vi "Step Make.vi"(8 "error in (no error)":errorcluster, 9 "Step Type (0: UP)":u16(ring) items=["Up", "Down"], 10 "Function (0: Voltage)":u16(ring) items=["Voltage", "Current"], 11 "VISA resource name":refnum<visa-resource-name>) -> (0 "error out":errorcluster, 3 "VISA resource name out":refnum<visa-resource-name>)   [LabVIEW 2015, in "IT6700H.lvlib"]
doc: "Change voltage or current value a step by UP and DOWN."
uses:
  <instrlib>/IT6700H/IT6700H.lvlib
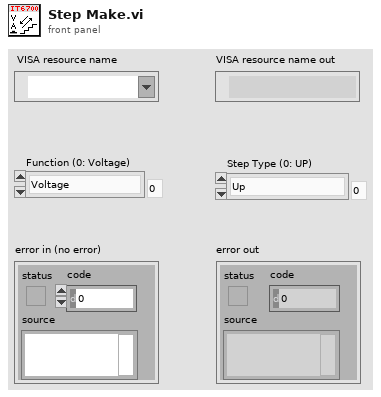
[diagram p1: front panel]
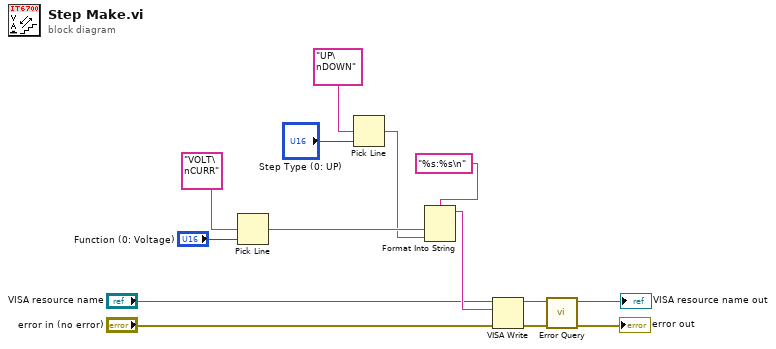
[diagram p0: block diagram]
diagram:
  n1 = Pick Line(multi-line string="VOLT\nCURR", line index="Function (0: Voltage)") -> (output string=w10:string)  [unwired: 1 in]
  n2 = Pick Line(multi-line string="UP\nDOWN", line index="Step Type (0: UP)") -> (output string=w9:string)  [unwired: 1 in]
  n3 = Format Into String(format string="%s:%s\n", w10, w9) -> (resulting string=w7:string)  [unwired: 2 in, 1 out]
  n4 = VISA Write(VISA resource name="VISA resource name", write buffer=w7, error in (no error)="error in (no error)") -> (VISA resource name out=w3:refnum<visa-resource-name>, error out=w4:errorcluster)  [unwired: 1 out]
  n5 = call <instrlib>:"Error Query.vi"("error in (no error)"=w4, "VISA resource name"=w3) -> ("error out"=→"error out":errorcluster, "VISA resource name out"=→"VISA resource name out":refnum<visa-resource-name>)  [unwired: 6 in, 2 out]
